vi "CRYStepSetup MNG.vi"(7 "sAction":string, 8 "nData":i32, 9 "sStepName":string, 10 "sOption":string, 11 "sData":string) -> (1 "pVIRef_Out":refnum<vi>, 3 "sData_Out":string)   [LabVIEW 2013]
uses:
  CRYStepSetup Global.vi
  CRYProject/CRYProject Editor Global.vi
panel:
  out "nData_Out":i32
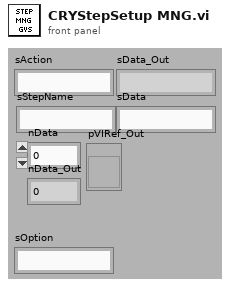
[diagram p1: front panel]
types:
  T1 = cluster{"nID":i32, "sName":string, "sType":string, "sProperty":string, "sTemplet":string, "sDocking":string, "pVIRef":refnum<vi>, "pSPRef":refnum<vi>, "pRefTemplet":refnum<vi>, "pRefSplitter":refnum<vi>[], "nPosSplitter":i32[], "pRefSP":refnum<vi>[], "nSPID":i32[], "sSPDock":string[], "nIDFrame":i32[], "nIDPanel":i32[], "nActiveFrame":i32, "nCountFrame":i32, "cFrame":cluster{"nID":i32, "sName":string, "sType":string, "sTitle":string, "sIcon":string, "pVIRef":refnum<vi>, "pSPRef":refnum<vi>, "cWiin":cluster{"sName":string, "sType":string, "pVIRef":refnum<vi>, "sData":string}, "cTab":cluster{"sTitle":string, "sIcon":string, "pSpliter":refnum<vi>, "nAvtivePage":i32, "nIDPage":i32[], "nIDFrame":i32[]}, "sData":string}[], "sData":string, "sSplitterName":string[]}
  T2 = typedef "CRYStep.ctl" = cluster{"No.VI":i32, "Category":string, "StepName":string, "Seq setup flattened":string, "Comment":string, "Steps config.":bool[], "Jump config":i32[], "Start":dbl, "Increment":dbl, "Name":string, "Unit":string, "Y data":u16, "Y prefix":string, "Y dB ref":dbl, "Y unit":string, "Repeat State Array":cluster{"Start":dbl, "Increment":dbl, "Count":i32, "Num":i32}[]}
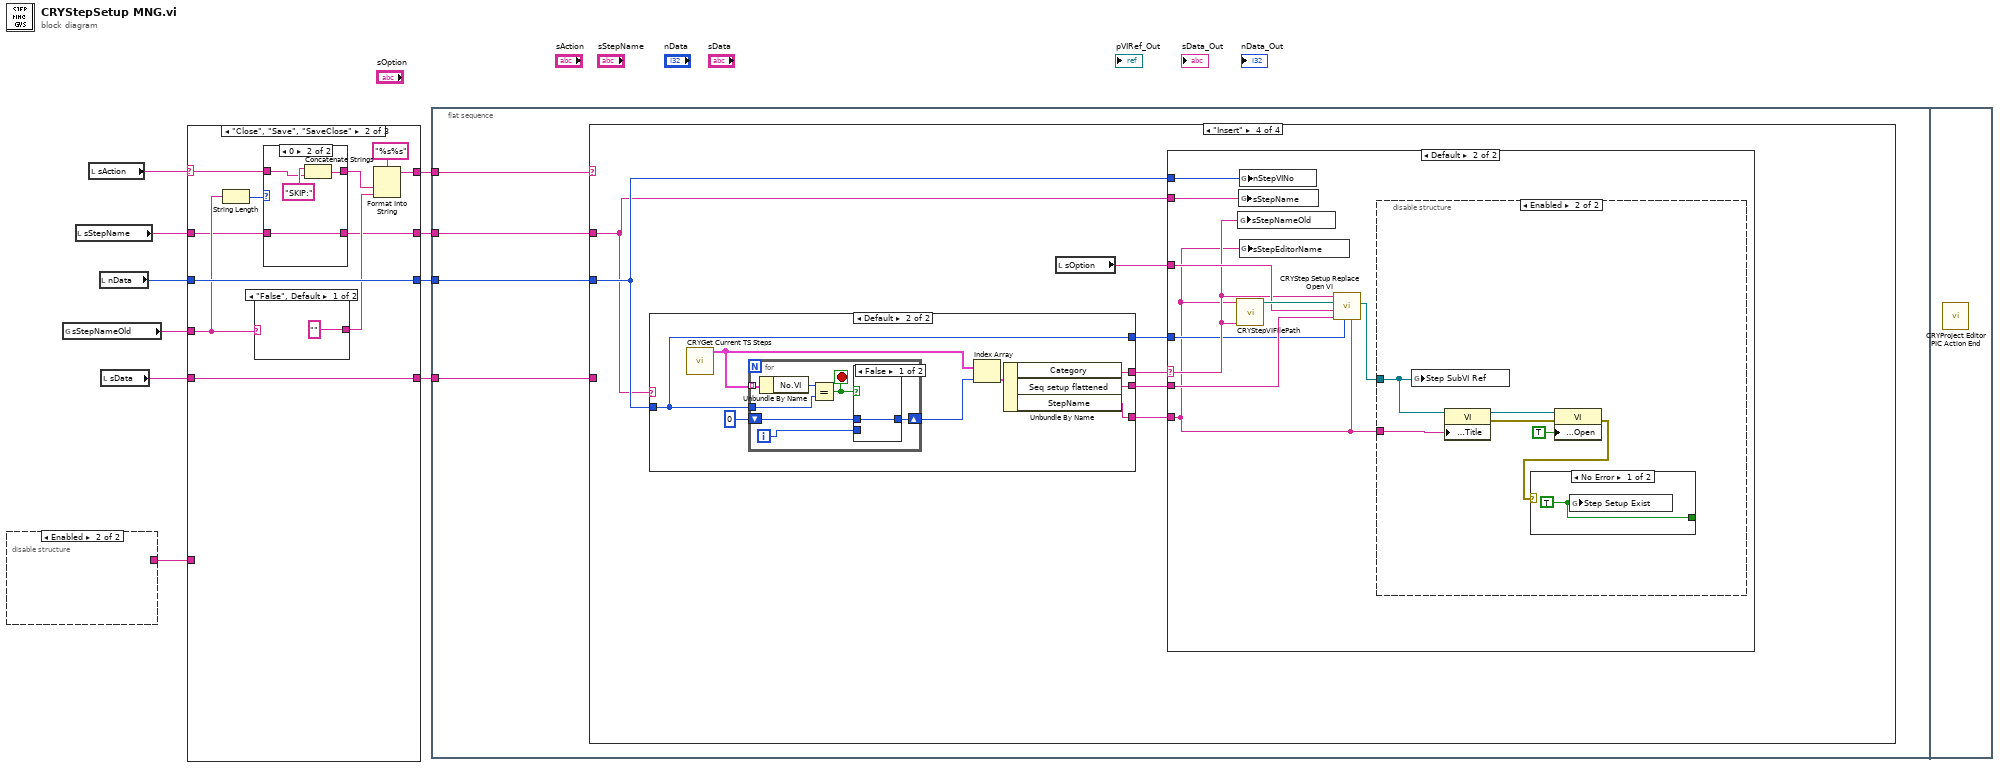
[diagram p0: block diagram]
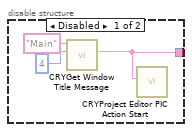
[diagram p2: hidden frame]
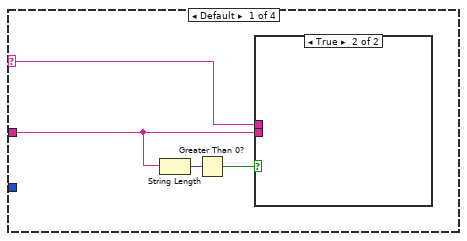
[diagram p3: hidden frame]
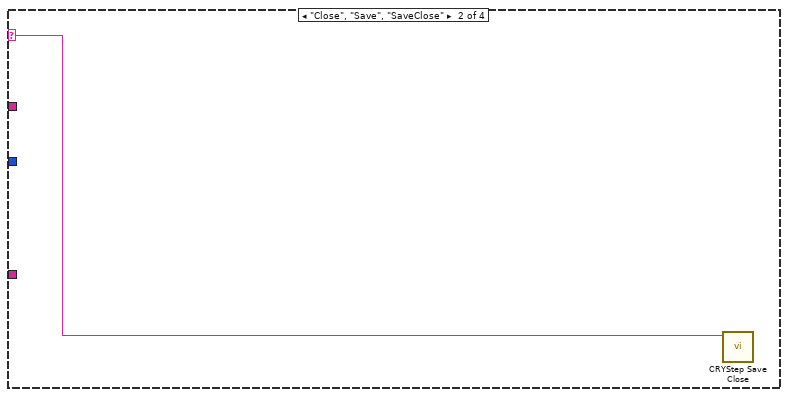
[diagram p5: hidden frame]
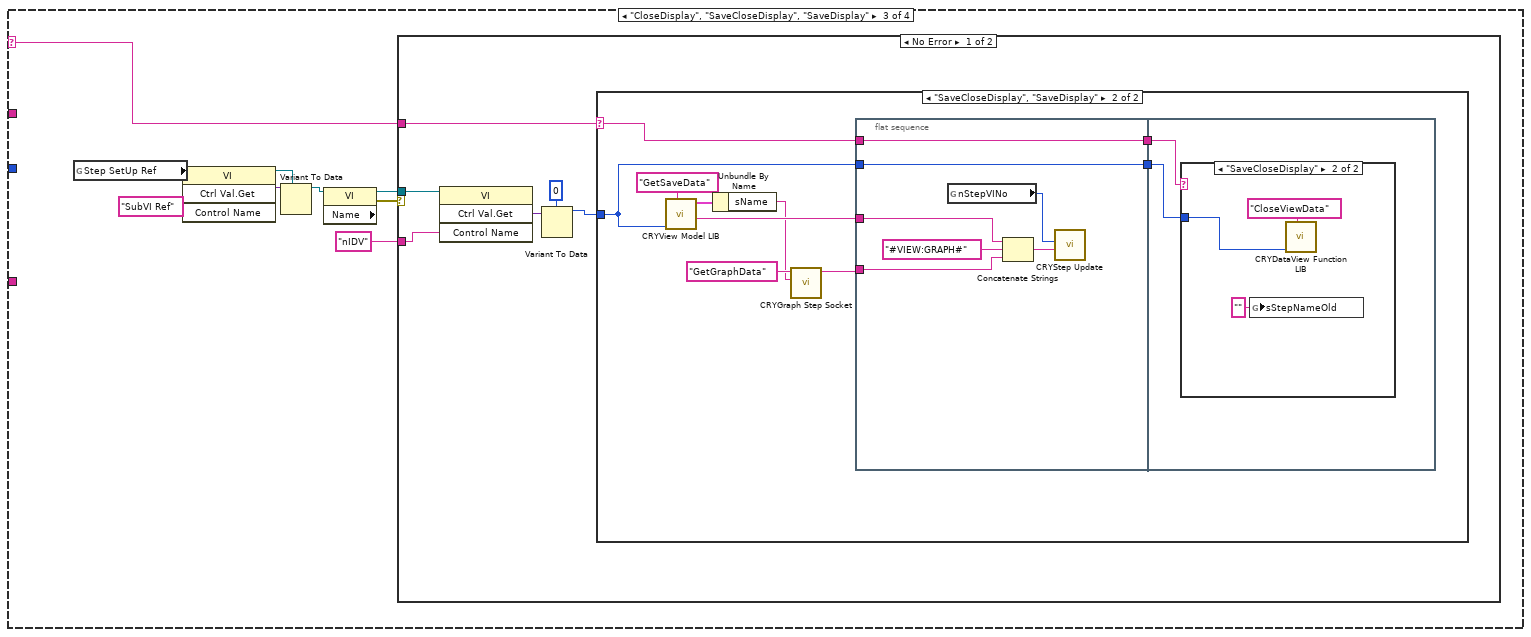
[diagram p6: hidden frame]
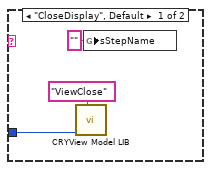
[diagram p7: hidden frame]
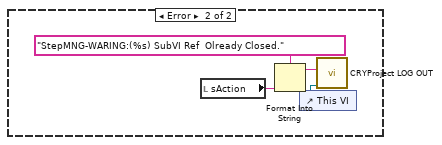
[diagram p9: hidden frame]
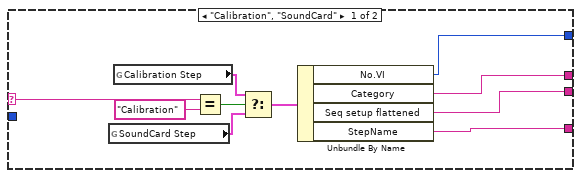
[diagram p10: hidden frame]
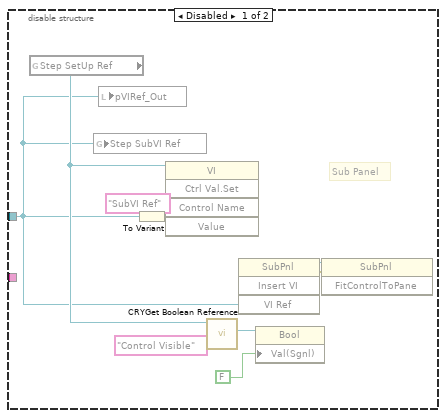
[diagram p13: hidden frame]
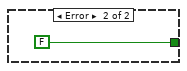
[diagram p14: hidden frame]
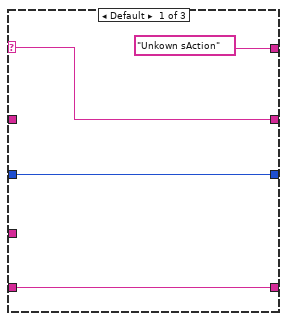
[diagram p15: hidden frame]
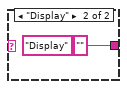
[diagram p17: hidden frame]
diagram:
  n1 = disable-structure shown="Enabled" {
    disable-tunnel: [w11 _] -> w1
    frame Disabled {
      n2 = call "CRYGet Window Title Message.vi"("No"=4, "Kind"="Main") -> ("Unicode String"=w11:string)  [unwired: 4 in, 5 out]
      n3 = call "CRYProject Editor PIC Action Start.vi"("sData"=w11) -> ()  [unwired: 11 in]
    }
    frame Enabled {
    }
  }
  n4 = global read "CRYStepSetup Global.vi" "sStepNameOld"() -> (w10:string)
  n5 = local read "sStepName"() -> (w9:string)
  n6 = local read "sAction"() -> (w2:string)
  n7 = local read "nData"() -> (w6:i32)
  n8 = local read "sData"() -> (w4:string)
  n9 = case shown="\"Close\", \"Save\", \"SaveClose\"" w2 {
    selector: w2 -> [w16 w22 w40]
    tunnel: w10 -> [_ w24 _]
    tunnel: w9 -> [_ w20 w39]
    tunnel: [w16 w19 w39] -> w7
    tunnel: ["Unkown sAction" ("format string") w27 w40] -> w8
    tunnel: w6 -> [w15 w26 w38]
    tunnel: [w15 w26 w38] -> w5
    tunnel: [w14 w18 w37] -> w3
    tunnel: w4 -> [w14 w18 w37]
    tunnel: w1 -> [_ _ _]
    frame Default {
    }
    frame "Close", "Save", "SaveClose" {
      n10 = String Length(string=w24) -> (length=w23:i32)
      n11 = case shown="\"False\", Default" w24 {
        tunnel: ["" ("sStepName") "" ("sStepName")] -> w25
        frame "False", Default {
        }
        frame "Display" {
          (unwired) "Display" ("sStepName")
        }
      }
      n12 = case shown="0" w23 {
        tunnel: w22 -> [w30 w32]
        tunnel: [w30 w34] -> w21
        tunnel: w20 -> [w29 w31]
        tunnel: [w29 w31] -> w19
        frame Default {
        }
        frame 0 {
          n13 = Concatenate Strings("SKIP:" ("format string"), w32) -> (w34:string)
        }
      }
      n14 = Format Into String(format string="%s%s", w21, w25) -> (resulting string=w27:string)  [unwired: 2 in, 1 out]
    }
    frame "Insert", "ReplaceDisplayStep" {
    }
  }
  n15 = flat-sequence {
    tunnel: w8 -> [w44]
    tunnel: w7 -> [w43]
    tunnel: w5 -> [w42]
    tunnel: w3 -> [w41]
    frame #0 {
      n16 = case shown="\"Insert\"" w44 {
        selector: w44 -> [w48 w49 w53 _]
        tunnel: w43 -> [w47 _ _ w96]
        tunnel: w42 -> [_ _ _ w100]
        tunnel: w41 -> [_ _ _ _]
        frame Default {
          n17 = String Length(string=w47) -> (length=w46:i32)
          n18 = Greater Than 0?(x=w46) -> (x > 0?=w45:bool)
          n19 = case shown="True" w45 {
            tunnel: w48 -> [_ _]
            tunnel: w47 -> [_ _]
            frame False {
            }
            frame True {
            }
          }
        }
        frame "Close", "Save", "SaveClose" {
          n20 = call "CRYStep Save Close.vi"("sAction"=w49) -> ()  [unwired: 11 in]
        }
        frame "CloseDisplay", "SaveCloseDisplay", "SaveDisplay" {
          n21 = global read "CRYStepSetup Global.vi" "Step SetUp Ref"() -> (w58:refnum<vi>)
          n22 = invoke class="VI" method="Ctrl Val.Get"(reference=w58, "Control Name"="SubVI Ref" ("Label Name")) -> (reference out=w56:refnum<vi>, "Get Control Value Variant"=w55:variant)  [unwired: 2 in, 2 out]
          n23 = Variant To Data(type=w56, Variant=w55) -> (data=w54:refnum<vi>)  [unwired: 1 in, 1 out]
          n24 = property class="VI" props=["Name"](reference=w54) -> (reference out=w51:refnum<vi>, error out=w52:errorcluster)  [unwired: 1 in, 1 out]
          n25 = case shown="No Error" w52 {
            tunnel: w53 -> [w62 _]
            tunnel: w51 -> [w61 _]
            tunnel: "nIDV" ("Control Name") -> [w60 _]
            frame No Error {
              n26 = invoke class="VI" method="Ctrl Val.Get"(reference=w61, "Control Name"=w60) -> ("Get Control Value Variant"=w64:variant)  [unwired: 2 in, 3 out]
              n27 = Variant To Data(type=0, Variant=w64) -> (data=w63:i32)  [unwired: 1 in, 1 out]
              n28 = case shown="\"SaveCloseDisplay\", \"SaveDisplay\"" w62 {
                selector: w62 -> [_ w77]
                tunnel: w63 -> [w65 w68]
                frame "CloseDisplay", Default {
                  n29 = call "CRYView Model LIB.vi"("sAction"="ViewClose", "nData"=w65) -> ()  [unwired: 7 in, 3 out]
                  n30 = global write "CRYStepSetup Global.vi" "sStepName"("" ("sStepName")) -> ()
                }
                frame "SaveCloseDisplay", "SaveDisplay" {
                  n31 = call "CRYView Model LIB.vi"("sAction"="GetSaveData", "nData"=w68) -> ("sData_Out"=w71:string, "cView_Out"=w70:T1)  [unwired: 7 in, 1 out]
                  n32 = Unbundle By Name(w70) -> ("sName"=w69:string)
                  n33 = call "CRYGraph Step Socket.vi"("Queue Name"=w69, "sAction"="GetGraphData") -> ("sDataOut"=w74:string)  [unwired: 9 in]
                  n34 = flat-sequence {
                    tunnel: w71 -> [w79]
                    tunnel: w68 -> [w84]
                    tunnel: w77 -> [w83]
                    tunnel: [w84] -> w76
                    tunnel: [w83] -> w75
                    tunnel: w74 -> [w78]
                    tunnel: w76 -> [w86]
                    tunnel: w75 -> [w85]
                    frame #0 {
                      n35 = global read "CRYStepSetup Global.vi" "nStepVINo"() -> (w82:i32)
                      n36 = Concatenate Strings(w79, "#VIEW:GRAPH#" ("regular expression"), w78) -> (w80:string)
                      n37 = call "CRYStep Update.vi"("Seq-step setup"=w80, "Proper VI No"=w82) -> ()  [unwired: 5 in, 5 out]
                    }
                    frame #1 {
                      n38 = case shown="\"SaveCloseDisplay\"" w85 {
                        tunnel: w86 -> [_ w88]
                        frame Default {
                        }
                        frame "SaveCloseDisplay" {
                          n39 = global write "CRYStepSetup Global.vi" "sStepNameOld"("" ("sStepName")) -> ()
                          n40 = call "CRYDataView Function LIB.vi"("sAction"="CloseViewData", "nData"=w88) -> ()  [unwired: 7 in, 3 out]
                        }
                      }
                    }
                  }
                }
              }
            }
            frame Error {
              n41 = local read "sAction"() -> (w90:string)
              n42 = Format Into String(format string="StepMNG-WARING:(%s) SubVI Ref  Olready Closed.", w90) -> (resulting string=w92:string)  [unwired: 2 in, 1 out]
              n43 = control-ref of="This VI"() -> (w93:refnum<vi>)
              n44 = call "CRYProject LOG OUT.vi"("pVIRef"=w93, "sData"=w92) -> ()  [unwired: 10 in]
            }
          }
        }
        frame "Insert" {
          n45 = case shown="Default" w96 {
            selector: w96 -> [w110 _]
            tunnel: w100 -> [_ w111]
            tunnel: [w103 w114] -> w99
            tunnel: [w104 w113] -> w98
            tunnel: [w102 w112] -> w95
            tunnel: [w101 w111] -> w94
            frame "Calibration", "SoundCard" {
              n46 = global read "CRYProject Editor Global.vi" "SoundCard Step"() -> (w105:T2)
              n47 = global read "CRYProject Editor Global.vi" "Calibration Step"() -> (w106:T2)
              n48 = Equal?(x=w110, y="Calibration") -> (x = y?=w108:bool)
              n49 = Select(t=w106, s=w108, f=w105) -> (s? t:f=w107:T2)
              n50 = Unbundle By Name(w107) -> ("No.VI"=w101:i32, "Category"=w104:string, "Seq setup flattened"=w103:string, "StepName"=w102:string)
            }
            frame Default {
              n51 = call "CRYGet Current TS Steps.vi"() -> ("Steps"=w117:T2[])  [unwired: 1 in, 10 out]
              n52 = for {
                tunnel: w117 -> [w125] mode=indexing
                tunnel: w111 -> [w123]
                shift-right: [w120] -> w116
                shift-left: 0 -> [w122]
                i -> [w119]
                stop <- w121 stop-if-true
                n53 = Unbundle By Name(w125) -> ("No.VI"=w124:i32)
                n54 = Equal?(x=w124, y=w123) -> (x = y?=w121:bool)
                n55 = case shown="False" w121 {
                  tunnel: w122 -> [w126 _]
                  tunnel: [w126 w127] -> w120
                  tunnel: w119 -> [_ w127]
                  frame False {
                  }
                  frame True {
                  }
                }
              }
              n56 = Index Array(array=w117, index=w116) -> (element=w115:T2)
              n57 = Unbundle By Name(w115) -> ("Category"=w113:string, "Seq setup flattened"=w114:string, "StepName"=w112:string)
            }
          }
          n58 = local read "sOption"() -> (w97:string)
          n59 = case shown="Default" w98 {
            selector: w98 -> [_ w130]
            tunnel: w96 -> [_ w131]
            tunnel: w100 -> [_ w135]
            tunnel: w99 -> [_ w134]
            tunnel: w97 -> [_ w132]
            tunnel: w95 -> [_ w128]
            tunnel: w94 -> [_ w129]
            frame "Display" {
            }
            frame Default {
              n60 = call "CRYStepVIFilePath.vi"("Category Name"=w130, "Step Name"=w128) -> ("Editor VI Path Out"=w136:path)  [unwired: 8 out]
              n61 = global write "CRYStepSetup Global.vi" "sStepNameOld"(w130) -> ()
              n62 = global write "CRYStepSetup Global.vi" "sStepName"(w131) -> ()
              n63 = global write "CRYStepSetup Global.vi" "nStepVINo"(w135) -> ()
              n64 = global write "CRYStepSetup Global.vi" "sStepEditorName"(w128) -> ()
              n65 = call "CRYStep Setup Replace Open VI.vi"("Step Name"=w128, "StepNo."=w129, "sData"=w134, "sOption"=w132, "VI Path"=w136, "Category"=w130) -> ("pVIRef"=w133:refnum<vi>)  [unwired: 4 in, 1 out]
              n66 = disable-structure shown="Enabled" {
                disable-tunnel: w133 -> [w137 w147]
                disable-tunnel: w128 -> [_ w150]
                frame Disabled {
                  # "Sub Panel"
                  n67 = global read "CRYStepSetup Global.vi" "Step SetUp Ref"() -> (w141:refnum<vi>)
                  n68 = global write "CRYStepSetup Global.vi" "Step SubVI Ref"(w137) -> ()
                  n69 = local write "pVIRef_Out"(w137) -> ()
                  n70 = To Variant(anything=w137) -> (Variant=w143:variant)
                  n71 = invoke class="VI" method="Ctrl Val.Set"(reference=w141, "Control Name"="SubVI Ref" ("Label Name"), "Value"=w143) -> ()  [unwired: 2 in, 5 out]
                  n72 = call "CRYGet Boolean Reference.vi"("Label Name"="Control Visible", "VI Refnum"=w141) -> ("Boolean Ref"=w145:refnum<vi>)  [unwired: 9 out]
                  n73 = invoke class="SubPnl" method="Insert VI"("VI Ref"=w137) -> (reference out=w139:refnum<vi>, error out=w138:errorcluster)  [unwired: 3 in, 2 out]
                  n74 = property class="Bool"(reference=w145, "Val(Sgnl)"=FALSE) -> ()  [unwired: 1 in, 2 out]
                  n75 = invoke class="SubPnl" method="FitControlToPane"(reference=w139, error in=w138) -> ()  [unwired: 1 in, 3 out]
                }
                frame Enabled {
                  n76 = global write "CRYStepSetup Global.vi" "Step SubVI Ref"(w147) -> ()
                  n77 = property class="VI"(reference=w147, "Front Panel.Title"=w150) -> (reference out=w149:refnum<vi>, error out=w148:errorcluster)  [unwired: 1 in]
                  n78 = property class="VI"(reference=w149, error in=w148, "Front Panel Window:Open"=TRUE ("Front Panel.Open")) -> (error out=w146:errorcluster)  [unwired: 1 out]
                  n79 = case shown="No Error" w146 {
                    tunnel: [w152 FALSE ("Step Setup Exist")] -> _
                    frame No Error {
                      w152 = TRUE ("Step Setup Exist")
                      n80 = global write "CRYStepSetup Global.vi" "Step Setup Exist"(w152) -> ()
                    }
                    frame Error {
                    }
                  }
                }
              }
            }
          }
        }
      }
    }
    frame #1 {
      n81 = call "CRYProject Editor PIC Action End.vi"() -> ()  [unwired: 12 in]
    }
  }
